vi "Write serialNumber.vi"(8 "error in (no error)":errorcluster, 10 "serialNumber":string, 11 "SCD in":refnum<class "SCD.lvclass">) -> (0 "error out":errorcluster, 3 "SCD out":refnum<class "SCD.lvclass">)   [LabVIEW 2023, in "horiba.lvlib" / "SCD.lvclass"]
doc: "Accessor VI for this class property."
uses:
  SCD.lvclass
  GenericDevice/GenericDevice.lvclass
  SCD.lvclass/SCD.ctl
panel:
  # "Connector Pane"
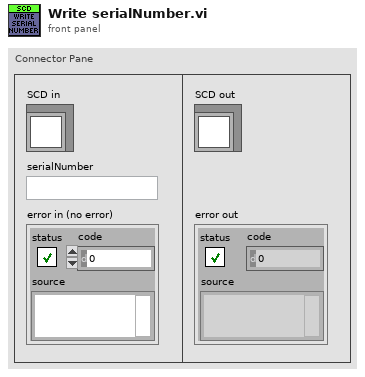
[diagram p1: front panel]
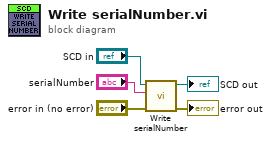
[diagram p0: block diagram]
diagram:
  n1 = call-parent "Write serialNumber.vi"("error in (no error)"="error in (no error)", "serialNumber"="serialNumber", "GenericDevice in"="SCD in") -> ("error out"=→"error out":errorcluster, "GenericDevice out"=→"SCD out":refnum<class "SCD.lvclass">)  [unwired: 7 in]
